vi "Get All Properties_3.vi"(8 "error in":errorcluster) -> (0 "error out":errorcluster, 3 "Properties[]":T1(array[cluster]))   [LabVIEW 2023]
panel:
  out "total class count":i32
  out "Classes processed":i32
  out "Class processing":string
  out "Property Ct":i32
  out "exe time (ms)":u32
  # "Original time was ca 5 min, improved class sorting and made sure we don't get properties for a class more than once:\n\n2504 props, 231 processed, 65s\n2504, 295 processed, 81s\n2504, 230 pricessed, 79s.\n\nLooks like sorting classes isn't needed\n\nNext round of improvement, pur helper VI refs in shift registers so we don't get class and proeprty node rein a loop\n\n2504, props, 25s. Wow!!!"
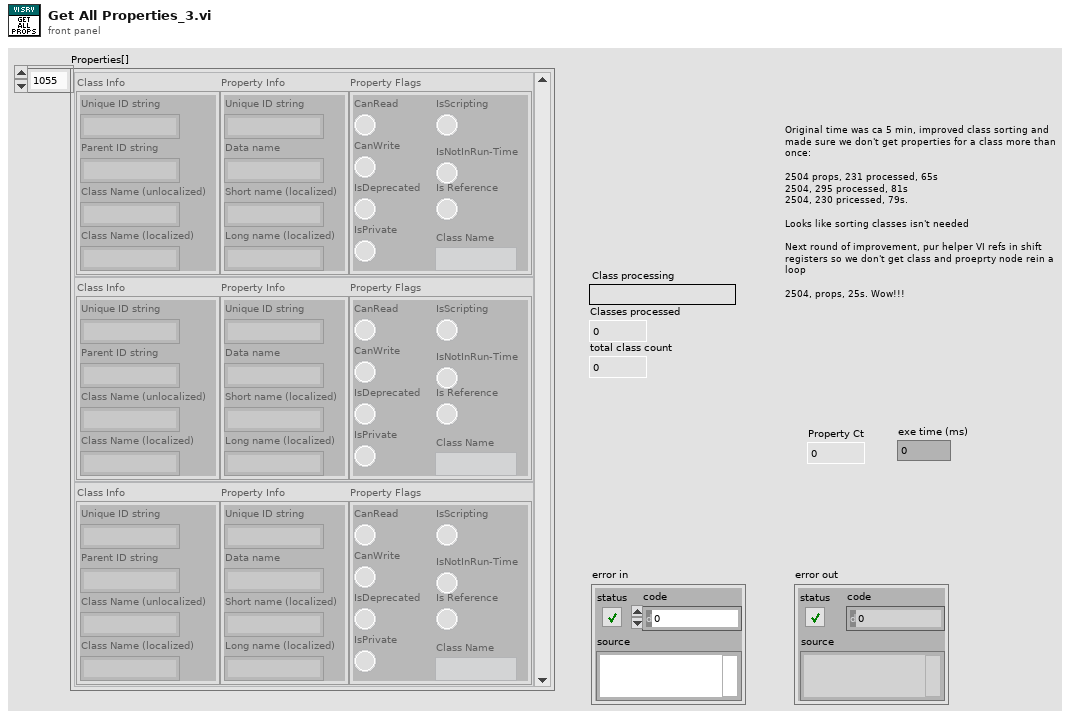
[diagram p1: front panel]
types:
  T1 = cluster{"Class Info":cluster{"Unique ID string":string, "Parent ID string":string, "Class Name (unlocalized)":string, "Class Name (localized)":string}, "Property Info":cluster{"Unique ID string":string, "Data name":string, "Short name (localized)":string, "Long name (localized)":string}, "Property Flags":cluster{"CanRead":bool, "CanWrite":bool, "IsDeprecated":bool, "IsPrivate":bool, "IsScripting":bool, "IsNotInRun-Time":bool, "Is Reference":bool, "Class Name":string}}[]
  T2 = cluster{"Unique ID string":string, "Parent ID string":string, "Class Name (unlocalized)":string, "Class Name (localized)":string}[]
  T3 = cluster{"Class Name":string, "Property Info":cluster{"Unique ID string":string, "Data name":string, "Short name (localized)":string, "Long name (localized)":string}}[]
  T4 = cluster{"Unique ID string":string, "Data name":string, "Short name (localized)":string, "Long name (localized)":string}
  T5 = cluster{"CanRead":bool, "CanWrite":bool, "IsDeprecated":bool, "IsPrivate":bool, "IsScripting":bool, "IsNotInRun-Time":bool, "Is Reference":bool, "Class Name":string}
  T6 = cluster{"Property/Method Info":cluster{"Unique ID string":string, "Parent ID string":string, "Class Name (unlocalized)":string, "Class Name (localized)":string}, "Property Info":cluster{"Unique ID string":string, "Data name":string, "Short name (localized)":string, "Long name (localized)":string}, "Property Flags":cluster{"CanRead":bool, "CanWrite":bool, "IsDeprecated":bool, "IsPrivate":bool, "IsScripting":bool, "IsNotInRun-Time":bool, "Is Reference":bool, "Class Name":string}}
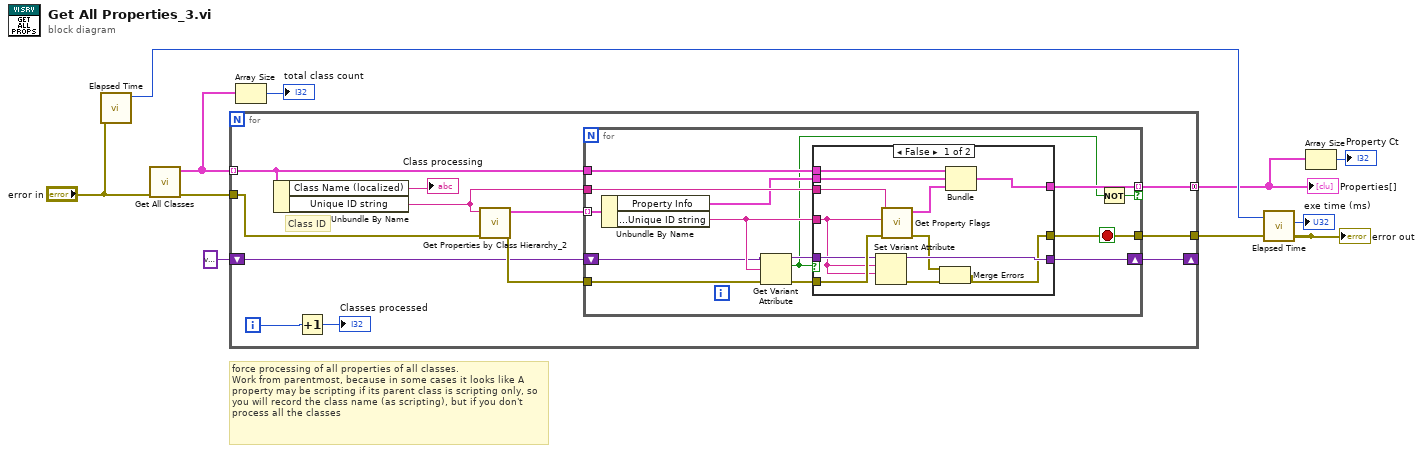
[diagram p0: block diagram]
diagram:
  # "force processing of all properties of all classes.\nWork from parentmost, because in some cases it looks like A property may be scripting if its parent class is scripting only, so you will record the class name (as scripting), but if you don't process all the classes"
  n1 = call "Elapsed Time.vi"("error in"="error in") -> ("millisecond timer value"=w8:u32)  [unwired: 7 in, 3 out]
  n2 = call "Get All Classes.vi"("error in (no error)"="error in") -> ("error out"=w10:errorcluster, "VI Server Classes[]"=w5:T2)  [unwired: 9 in]
  n3 = for {
    tunnel: w10 -> [w22]
    tunnel: [w13] -> w1
    shift-right: [w19] -> _
    shift-left: variant -> [w18]
    tunnel: [w16] -> w2 mode=concatenating
    tunnel: w5 -> [w11] mode=indexing
    i -> [w15]
    # "Class ID"
    n4 = Unbundle By Name(w11) -> ("Class Name (localized)"=→"Class processing":string, "Unique ID string"=w17:string)
    n5 = Increment(x=w15) -> (x+1=→"Classes processed":i32)
    n6 = call "Get Properties by Class Hierarchy_2.vi"("error in (no error)"=w22, "Class ID"=w17) -> ("error out"=w21:errorcluster, "Properties by Class Hierarchy"=w20:T3)  [unwired: 7 in, 1 out]
    n7 = for {
      tunnel: w20 -> [w25] mode=indexing
      tunnel: w11 -> [w27]
      tunnel: w21 -> [w35]
      tunnel: [w36] -> w13
      shift-right: [w32] -> w19
      shift-left: w18 -> [w31]
      tunnel: w17 -> [w29]
      tunnel: [w28] -> w16 mode=indexing if=w23
      stop <- w36 stop-if-true
      n8 = Unbundle By Name(w25) -> ("Property Info"=w26:T4, "Property Info.Unique ID string"=w33:string)
      n9 = Get Variant Attribute(Variant=w31, name=w33, error in=w35) -> (duplicate Variant=w30:variant, found=w24:bool, error out=w34:errorcluster)  [unwired: 1 in, 1 out]
      n10 = case shown="False" w24 {
        tunnel: w29 -> [w37 _]
        tunnel: w27 -> [w48 _]
        tunnel: [w38 w50] -> w36
        tunnel: w26 -> [w47 _]
        tunnel: w34 -> [w46 w50]
        tunnel: w33 -> [w41 _]
        tunnel: [w44 w49] -> w32
        tunnel: w30 -> [w43 w49]
        tunnel: [w42 _] -> w28
        frame False {
          n11 = Set Variant Attribute(Variant=w43, name=w41, value=w41) -> (Variant out=w44:variant, error out=w40:errorcluster)  [unwired: 1 in, 1 out]
          n12 = call "Get Property Flags.vi"("error in (no error)"=w46, "Property ID"=w41, "Class ID"=w37) -> ("error out"=w39:errorcluster, "Property Flags"=w45:T5)  [unwired: 7 in]
          n13 = Merge Errors(w39, w40) -> (w38:errorcluster)
          n14 = Bundle("Property/Method Info"=w48, "Property Info"=w47, "Property Flags"=w45) -> (w42:T6)  [unwired: 1 in]
        }
        frame True {
        }
      }
      n15 = Not(x=w24) -> (.not. x?=w23:bool)
    }
  }
  "Properties[]" <- w2
  "error out" <- w1
  n16 = Array Size(array=w5) -> (size(s)=→"total class count":i32)
  n17 = call "Elapsed Time.vi"("error in"=w1, "past time"=w8) -> ("elapsed time (ms)"=→"exe time (ms)":u32)  [unwired: 6 in, 3 out]
  n18 = Array Size(array=w2) -> (size(s)=→"Property Ct":i32)
